vi "generaAleatorio.vi"(2 "Parametros Maximos":T1, 3 "Sound Parameters":cluster{"# samples":u32, "tiempos (ms)":dbl}, 4 "Señal de Control IN":dbl[](array[numeric])) -> (0 "Parametros Iniciales":T1, 1 "Out":dbl[](array[numeric]))   [LabVIEW 2010]
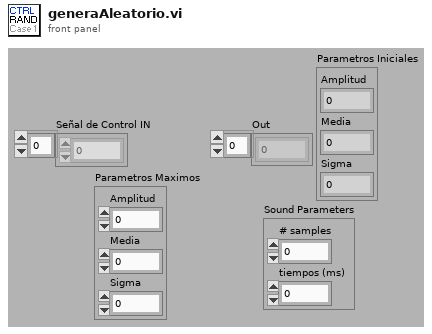
[diagram p1: front panel]
types:
  T1 = cluster{"Amplitud":dbl, "Media":dbl, "Sigma":dbl}
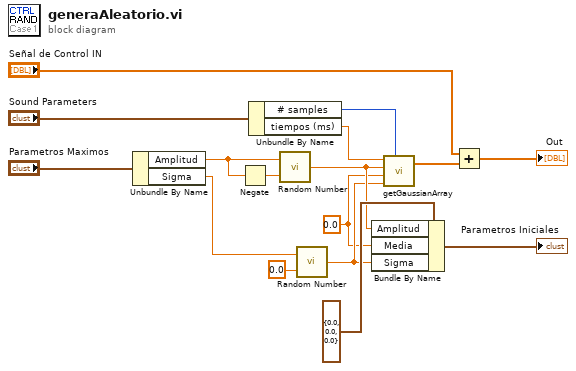
[diagram p0: block diagram]
diagram:
  w1 = 0.0 ("t0 (ms)")
  n1 = Unbundle By Name("Parametros Maximos") -> ("Amplitud"=w8:dbl, "Sigma"=w7:dbl)
  n2 = Negate(x=w8) -> (-x=w12:dbl)
  n3 = Unbundle By Name("Sound Parameters") -> ("# samples"=w5:u32, "tiempos (ms)"=w4:dbl)
  n4 = call "Random Number.vi"("Min"=w12, "Max"=w8) -> ("Out"=w3:dbl)
  n5 = call "Random Number.vi"("Min"=0.0, "Max"=w7) -> ("Out"=w2:dbl)
  n6 = Bundle By Name(cluster=T1 {"Amplitud"=0.0, "Media"=0.0, "Sigma"=0.0} ("input cluster"), "Amplitud"=w3, "Media"=w1, "Sigma"=w2) -> (→"Parametros Iniciales":T1)
  n7 = call "getGaussianArray.vi"("tiempo (ms)"=w4, "Amplitud"=w3, "t0 (ms)"=w1, "Sigma (ms)"=w2, "#samples"=w5) -> ("Y out"=w15:dbl[])  [unwired: 1 out]
  n8 = Add(x="Señal de Control IN", y=w15) -> (x+y=→"Out":dbl[])
